vi "Get Error Message.vi"(8 "error in (no error)":errorcluster, 11 "SQL Statement In":refnum<class "SQL Statement.lvclass">) -> (0 "error out":errorcluster, 2 "error message":string, 3 "SQL Statement Out":refnum<class "SQL Statement.lvclass">)   [LabVIEW 2023, in "SQLite.lvlib" / "SQL Statement.lvclass"]
uses:
  SQL Statement.lvclass
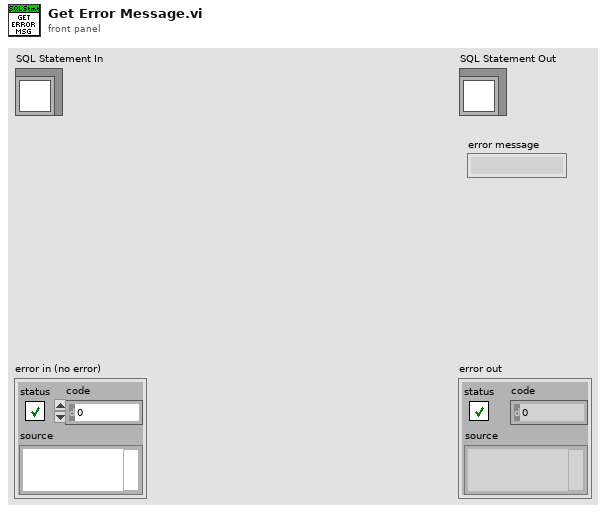
[diagram p1: front panel]
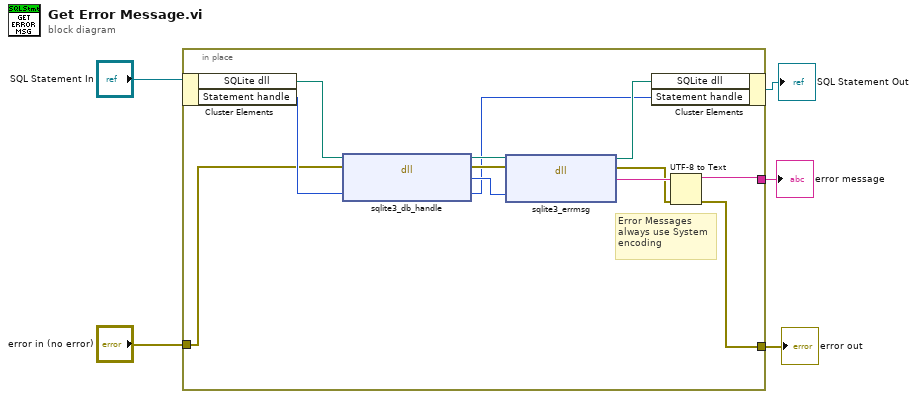
[diagram p0: block diagram]
diagram:
  n1 = in-place {
    in-place-border: "error in (no error)" -> [w10]
    in-place-border: [w6] -> w4
    in-place-border: [w8] -> w3
    # "Error Messages\nalways use System\nencoding"
    n2 = in-place-cluster #1("SQL Statement In") -> ("SQLite dll"=w11:path, "Statement handle"=w12:u64)
    n3 = dll-call lib="C:/LabVIEW_JDP/Support/SQLite/SQL Connection/sqlite3.dll" fn="sqlite3_db_handle"(path in=w11, error in=w10, "stmt handle"=w12) -> (path out=w16:path, error out=w15:errorcluster, "db handle"=w14:u64, "stmt handle"=w13:u64)  [unwired: 1 in]
    n4 = dll-call lib="C:/LabVIEW_JDP/Support/SQLite/SQL Connection/sqlite3.dll" fn="sqlite3_errmsg"(path in=w16, error in=w15, "db handle"=w14) -> (path out=w17:path, error out=w7:errorcluster, "error message"=w9:string)  [unwired: 2 in]
    n5 = in-place-cluster #1("SQLite dll"=w17, "Statement handle"=w13) -> (→"SQL Statement Out":refnum<class "SQL Statement.lvclass">)
    n6 = UTF-8 to Text(8:w7, 11:w9) -> (0:w6:errorcluster, 3:w8:string)  [unwired: 1 in]
  }
  "error out" <- w4
  "error message" <- w3
